vi "Read Session ID.vi"(8 "error in (no error)":errorcluster, 11 "Session in":refnum<class "Session.lvclass">) -> (0 "error out":errorcluster, 2 "Session ID":i32, 3 "Session out":refnum<class "Session.lvclass">)   [LabVIEW 2013, in "MQTT Server.lvlib" / "Session.lvclass"]
uses:
  Session.lvclass
  Session.lvclass/Session.ctl
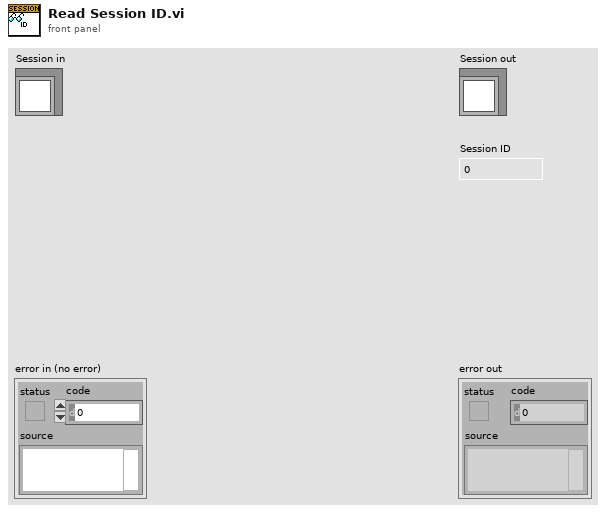
[diagram p1: front panel]
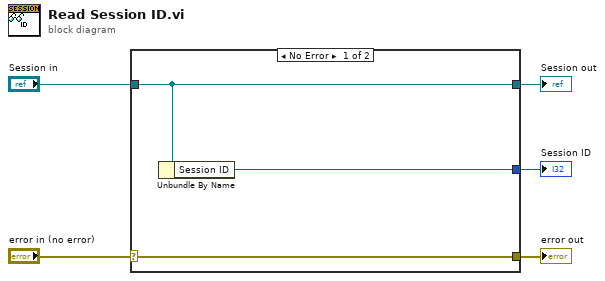
[diagram p0: block diagram]
diagram:
  n1 = case shown="No Error" "error in (no error)" {
    selector: "error in (no error)" -> [w8 w9]
    tunnel: [w8 w9] -> w4
    tunnel: [w7 w10] -> w2
    tunnel: "Session in" -> [w7 w10]
    tunnel: [w6 _] -> w1
    frame No Error {
      n2 = Unbundle By Name(w7) -> ("Session ID"=w6:i32)
    }
    frame Error {
    }
  }
  "error out" <- w4
  "Session out" <- w2
  "Session ID" <- w1
